vi "myYield.vi"() -> ()   [LabVIEW 2018]
uses:
  <vilib>/addons/Tools/Unicode/UTF8 Tools.lvlib
panel:
  out "Consecutive Fails":dbl
  out "error out":errorcluster
  in  "error in (no error)":errorcluster
  out "Cluster":T1
  out "Return Code":i64
  out "Python Output":string
  in  "Path of Log":path
  out "Fails":dbl
  out "Passes":dbl
  out "Total Tests":dbl
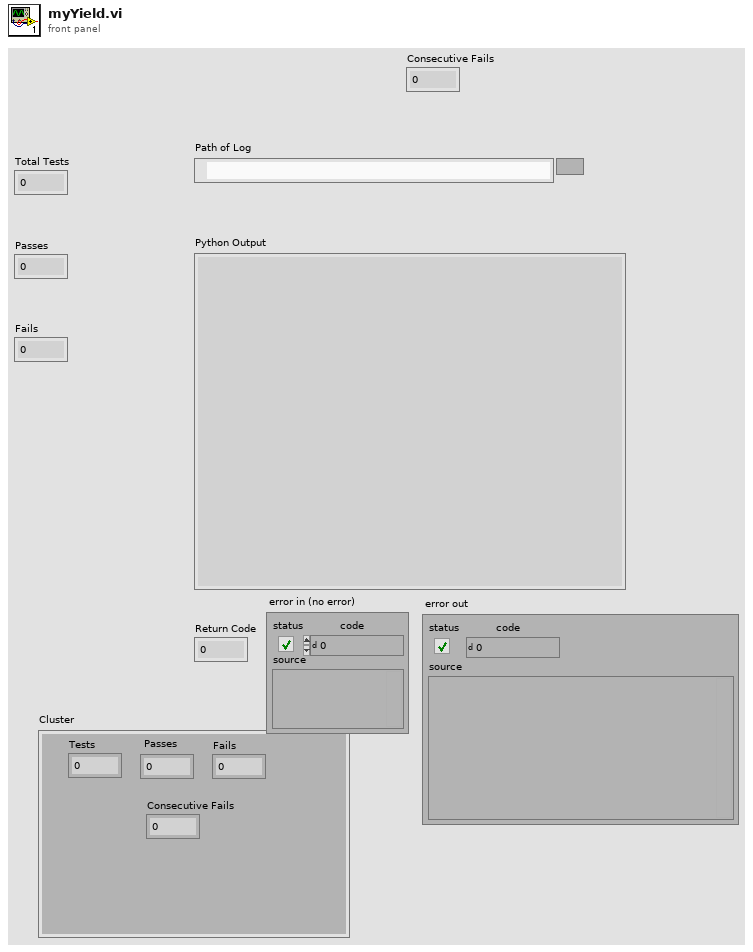
[diagram p1: front panel]
types:
  T1 = cluster{"Tests":i32, "Passes":i32, "Fails":i32, "Consecutive Fails":i32}
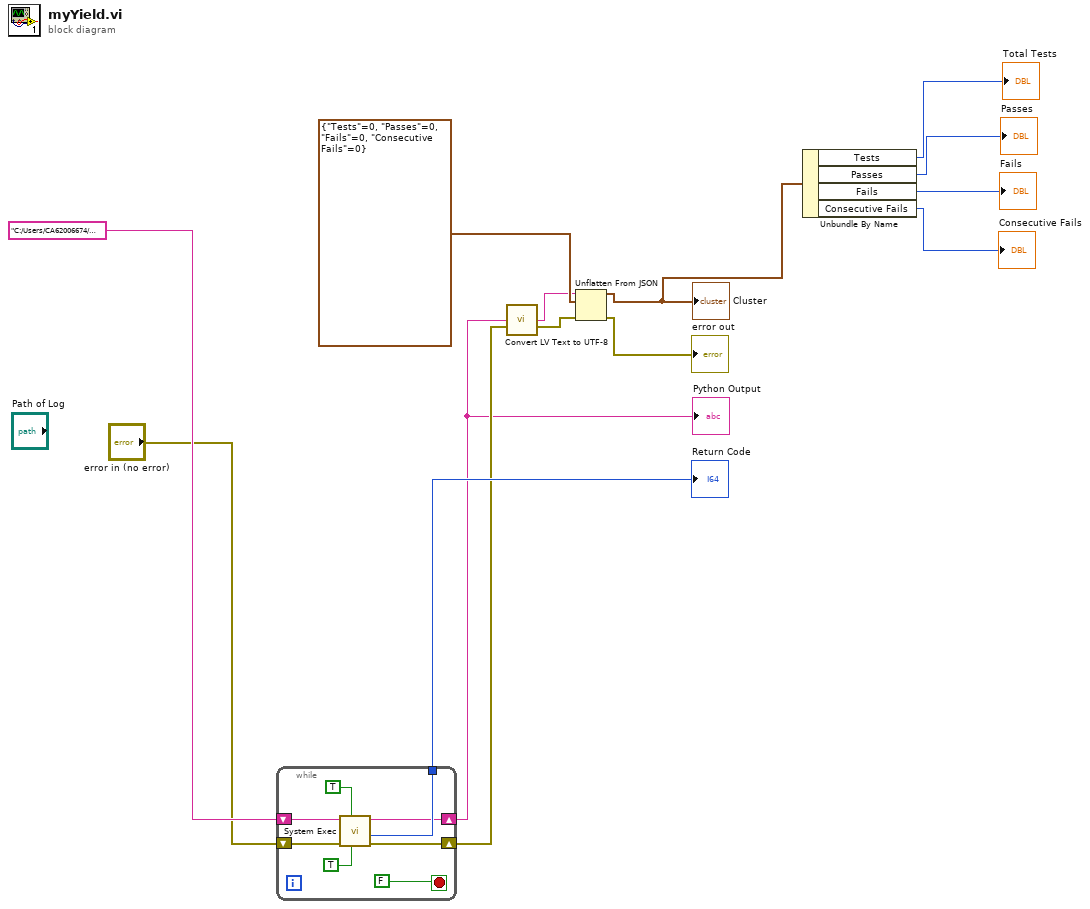
[diagram p0: block diagram]
diagram:
  n1 = while {
    tunnel: [w21] -> w13
    shift-right: [w17] -> w6
    shift-left: "C:/Users/CA62006674/AppData/Local/Programs/Python/Python37/python.exe c:/Users/CA62006674/Desktop/myPythonPractice/myYieldTool.py c:/Users/CA62006674/Desktop/myPythonPractice" -> [w22]
    shift-right: [w19] -> w9
    shift-left: "error in (no error)" -> [w20]
    stop <- FALSE stop-if-true
    n2 = call <vilib>:"System Exec.vi"("run minimized? (F)"=TRUE, "wait until completion? (T)"=TRUE, "error in (no error)"=w20, "command line"=w22) -> ("error out"=w19:errorcluster, "return code"=w21:i32, "standard output"=w17:string)  [unwired: 4 in, 1 out]
  }
  "Python Output" <- w6
  "Return Code" <- w13
  n3 = call <vilib>:"Convert LV Text to UTF-8.vi"("LV Text"=w6, "error in"=w9) -> ("UTF-8 Text"=w11:string, "error out"=w8:errorcluster)  [unwired: 12 in]
  n4 = Unflatten From JSON(JSON string=w11, type and defaults=T1 {"Tests"=0, "Passes"=0, "Fails"=0, "Consecutive Fails"=0}, error in (no error)=w8) -> (value=w5:T1, error out=→"error out":errorcluster)  [unwired: 4 in]
  "Cluster" <- w5
  n5 = Unbundle By Name(w5) -> ("Tests"=→"Total Tests":i32, "Passes"=→"Passes":i32, "Fails"=→"Fails":i32, "Consecutive Fails"=→"Consecutive Fails":i32)
